vi "Execute Command Line With Switches FileIO.vi"(6 "Add Command Quotes?":bool, 7 "wait until completion? (T)":bool=TRUE, 8 "error in (no error)":errorcluster, 9 "Command Line Switches":string[](array[string]), 10 "Command (dir)":string="dir", 11 "Application Path":path) -> (0 "error out":errorcluster, 3 "Standard Output":string)   [LabVIEW 2015]
doc: "This VI will run a command line call similar to the Run function in Windows. Enter the <B>Application Path</B> to be executed or enter it in as the <B>Command (dir)</B>. Optionally <B>Command Line Switches</B> can be passed to the application. These will be space delimited commands.\n\nFor example to copy a file from a location to another enter <B>copy</B> into the <B>Command</B> and <B>C:\\Program Files\\file1.txt</B> and <B>C:\\Program Files (x86)\\file1.txt</B> into the <B>Command Line Switches</B> to copy the file.\n\n-----\nBrian Hoover (Hooovahh)"
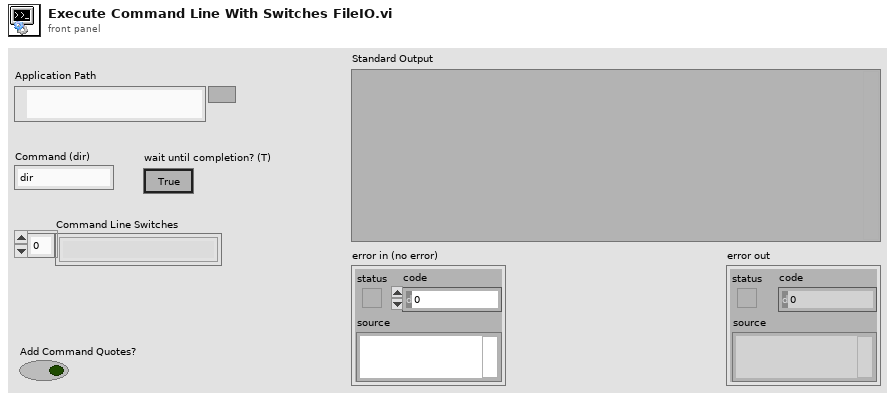
[diagram p1: front panel]
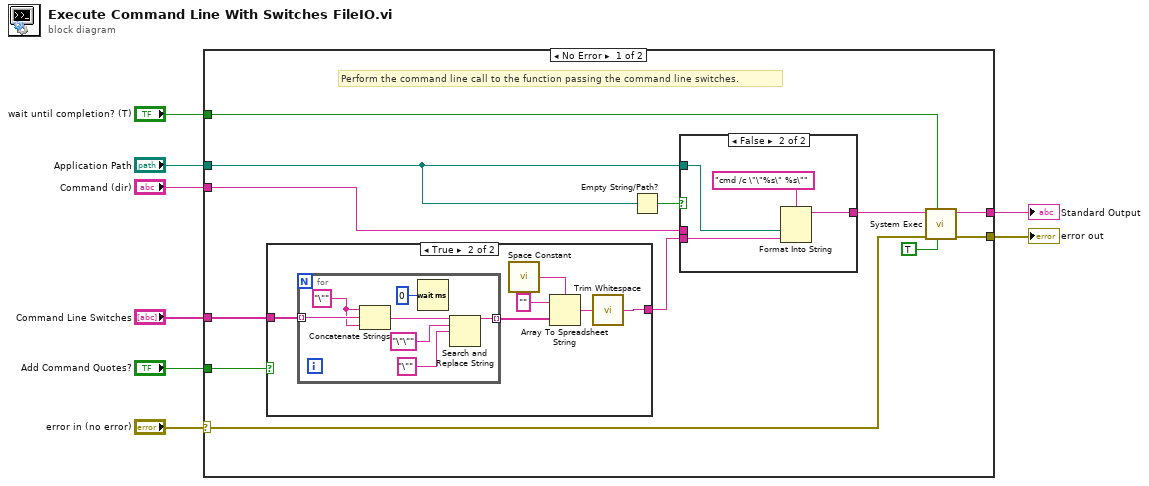
[diagram p0: block diagram]
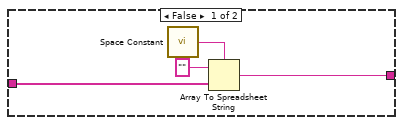
[diagram p2: hidden frame]
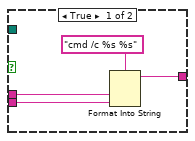
[diagram p3: hidden frame]
diagram:
  n1 = case shown="No Error" "error in (no error)" {
    selector: "error in (no error)" -> [w10 w46]
    tunnel: [w20 _] -> w8
    tunnel: "Command Line Switches" -> [w18 _]
    tunnel: "Command (dir)" -> [w17 _]
    tunnel: "Application Path" -> [w13 _]
    tunnel: [w12 w46] -> w4
    tunnel: "Add Command Quotes?" -> [w11 _]
    tunnel: "wait until completion? (T)" -> [w9 _]
    frame No Error {
      # "Perform the command line call to the function passing the command line switches."
      n2 = case shown="True" w11 {
        tunnel: w18 -> [w22 w27]
        tunnel: [w21 w25] -> w16
        frame False {
          n3 = call <vilib>:"Space Constant.vi"() -> ("String"=w23:string)
          n4 = Array To Spreadsheet String(delimiter (Tab)=w23, array=w22, 3:"" ("format string")) -> (spreadsheet string=w21:string)
        }
        frame True {
          n5 = for {
            tunnel: w27 -> [w37] mode=indexing
            tunnel: [w31] -> w26 mode=indexing
            w36 = "\"" ("string")
            n6 = Concatenate Strings(w36, w37, w36) -> (w35:string)
            n7 = Wait (ms)(milliseconds to wait=u32 0) -> ()  [unwired: 1 out]
            n8 = Search and Replace String(input string=w35, search string="\"\"", replace string="\"" ("replace string (\"\")")) -> (result string=w31:string)  [unwired: 5 in, 3 out]
          }
          n9 = call <vilib>:"Space Constant.vi"() -> ("String"=w29:string)
          n10 = Array To Spreadsheet String(delimiter (Tab)=w29, array=w26, 3:"" ("format string")) -> (spreadsheet string=w28:string)
          n11 = call <vilib>:"Trim Whitespace.vi"("string"=w28) -> ("trimmed string"=w25:string)  [unwired: 1 in]
        }
      }
      n12 = Empty String/Path?(string/path=w13) -> (empty?=w14:bool)
      n13 = case shown="False" w14 {
        tunnel: w17 -> [w40 _]
        tunnel: w16 -> [w39 w44]
        tunnel: [w38 w43] -> w15
        tunnel: w13 -> [_ w42]
        frame True {
          n14 = Format Into String(format string="cmd /c %s %s", w40, w39) -> (resulting string=w38:string)  [unwired: 2 in, 1 out]
        }
        frame False {
          n15 = Format Into String(format string="cmd /c \"\"%s\" %s\"", w42, w44) -> (resulting string=w43:string)  [unwired: 2 in, 1 out]
        }
      }
      n16 = call <vilib>:"System Exec.vi"("run minimized? (F)"=TRUE, "wait until completion? (T)"=w9, "error in (no error)"=w10, "command line"=w15) -> ("error out"=w12:errorcluster, "standard output"=w20:string)  [unwired: 4 in, 2 out]
    }
    frame Error {
    }
  }
  "Standard Output" <- w8
  "error out" <- w4
